vi "9149 FPGA VI.vi"() -> ()   [LabVIEW 2017]
uses:
  <vilib>/Platform/TimedLoop/XDataNode/timing_clust.ctl
  <vilib>/Platform/TimedLoop/XDataNode/nitl_modes.ctl
  <vilib>/Platform/TimedLoop/XDataNode/wakeup.ctl
  <vilib>/rvi/Emulation/niFpgaGetClockAttributes.vi
  <vilib>/rvi/Emulation/niFpgaSctlEmulationGetInTimedLoop.vi
  <vilib>/rvi/Emulation/niFpgaEmulationReportErrorSimple.vi
  <vilib>/rvi/eio/common/nirviEmuTemplateMethod_errors.vi
  <vilib>/rvi/Emulation/niFpgaEmulationIsFPGAContextNoSignature.vi
  <vilib>/rvi/errors/niFpgaSetErrorForExecOnDevCompSimple.vi
  <vilib>/rvi/eio/common/nirviEmuReportErrorAndStop.vi
  <vilib>/rvi/DataTransferAndStorage/Container/Common/niFpgaContainerGetUniqueNameForEmu.vi
  <vilib>/rvi/FIFO/Fifo_Resource/nirvififoEmulationSetSize.vi
  <vilib>/rvi/FIFO/Fifo_Resource/nirviFifoEmulationQueueMgr.vi
  <instcachedir>/0/nirviFifoEmulationQueueMgr_E5CAEC123FF24DC58D834DCA3CDAA9B5.lvgen/nirviFifoEmulationQueueMgr_E5CAEC123FF24DC58D834DCA3CDAA9B5_008.vi
  <vilib>/rvi/FIFO/Fifo_Resource/nirvififoEmulationDetermineInputValidOut.vi
  <vilib>/rvi/FIFO/Fifo_Resource/nirvififoEmulationCreateLock.vi
  <vilib>/rvi/Emulation/niFpgaProcessEmulError.vi
  <vilib>/rvi/FIFO/Fifo_Resource/nirvififoEmulationObtainLock.vi
  <vilib>/rvi/FIFO/Fifo_Resource/nirvififoEmulationReleaseLock.vi
  <vilib>/rvi/occurrence/nirviWaitOnOccurrenceBase.vi
  <vilib>/rvi/errors/nirviReportUnexpectedCaseInternalError.vi
  <vilib>/rvi/errors/nirviReportUnexpectedCaseInternalError (U32).vi
  <vilib>/rvi/Emulation/niFpgaCriticalErrorInLSC.vi
  <vilib>/Utility/error.llb/Clear Errors.vi
  <vilib>/rvi/interface/RandomDataEmulation/niFpgaRandomDataHandleErrors.vi
  <vilib>/eio/EIONode/EIONode.xnode
  <vilib>/rvi/DataTransferAndStorage/Container/XNode/niFpgaContainer.xnode
  <vilib>/rvi/FIFO/Fifo_Resource/nirvififoEmulationWrite.vi
  <vilib>/Platform/TimedLoop/XDataNode/XDataNode.xnode
  <vilib>/rvi/FIFO/Fifo_Resource/nirvififoEmulationRead.vi
  <vilib>/rvi/interface/RandomDataEmulation/nirviRandomDataFpgaReadWriteTemplate.vi
  <vilib>/Platform/TimedLoop/XDataNode/XDNodeRunTimeDep.lvlib
panel:
  out "Mod3_AI15_I32":i32
  out "Mod3_AI14_I32":i32
  out "Mod3_AI13_I32":i32
  out "Mod3_AI12_I32":i32
  out "Mod3_AI11_I32":i32
  out "Mod3_AI10_I32":i32
  out "Mod3_AI9_I32":i32
  out "Mod3_AI8_I32":i32
  out "Mod3_AI7_I32":i32
  out "Mod3_AI6_I32":i32
  out "Mod3_AI5_I32":i32
  out "Mod3_AI4_I32":i32
  out "TargetToHostLoopIterCount":i32
  out "TargetToHostLoopTimedOut":bool
  out "Mod6_U32":u32
  in  "Mod1_U32":u32
  in  "SlowDOLoop_Rate_us":u32=10000 caption="Count(uSec)"
  out "SlowDOLoop_Duration_ticks":u32
  in  "FastAILoop_Rate_us":u32=1000 caption="Count(uSec)"
  out "FastAILoop_Duration_ticks":u32
  out "Mod3_AI3_I32":i32
  out "Mod3_AI2_I32":i32
  out "Mod3_AI1_I32":i32
  out "Mod3_AI0_I32":i32
  out "SlowScanLoopTimedOut":bool
  out "SlowScanLoop_Duration_ticks":u32
  in  "SlowScanLoop_Rate_us":u32=10000 caption="Count(uSec)"
  in  "FastDO_Mod5_U8":u8
  out "FastDI_Mod8_U8":u8
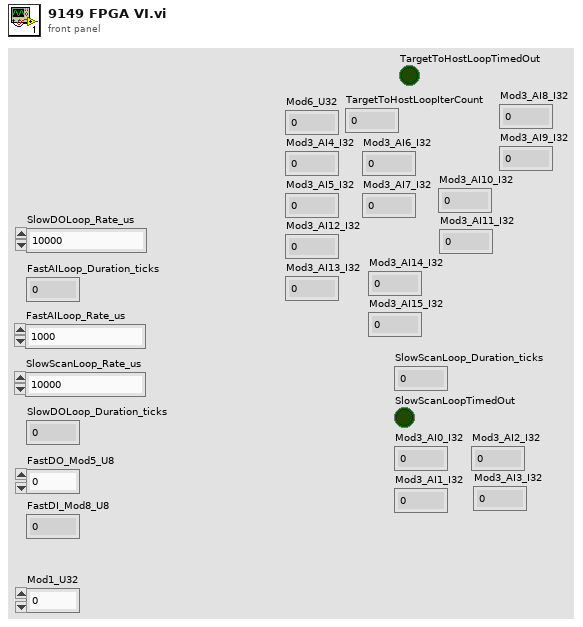
[diagram p1: front panel]
types:
  T1 = typedef "XDNodeRunTimeDep.lvlib/timing_clust.ctl" = cluster{"Expected End [f-1]":u64, "Actual End [f-1]":u64, "Finished Late? [f-1]":bool, "Expected End [i-1]":u64, "Actual End [i-1]":u64, "Finished Late? [i-1]":bool, "Expected Start [i]":u64, "Actual Start [i]":u64, "Expected Start [f]":u64, "Actual Start [f]":u64, "Source Name":string, "Structure Name":string, "Period":i64, "Deadline":i64, "Offset":i64, "Start":i64, "Priority":i32, "Timeout":i32, "Mode":T2, "Wakeup Reason":T3, "Error":errorcluster, "Source Type":string, "Secondary Source Type":string, "Global End Time":u64, "Global Start Time":u64, "Frame Duration":u64, "Iteration Duration":u64, "Assigned CPU":i32, "I/O Scan Engine Mode":u32}
  T2 = typedef "XDNodeRunTimeDep.lvlib/nitl_modes.ctl" = enum32{"No Change", "Process missed periods, maintain original phase", "Discard missed periods, maintain original phase", "Process missed periods, ignore original phase", "Discard missed periods, ignore original phase"}
  T3 = typedef "XDNodeRunTimeDep.lvlib/wakeup.ctl" = enum32{"Normal", "Aborted", "Asynchronous wakeup", "Timing source error", "Timed loop error", "Timeout"}
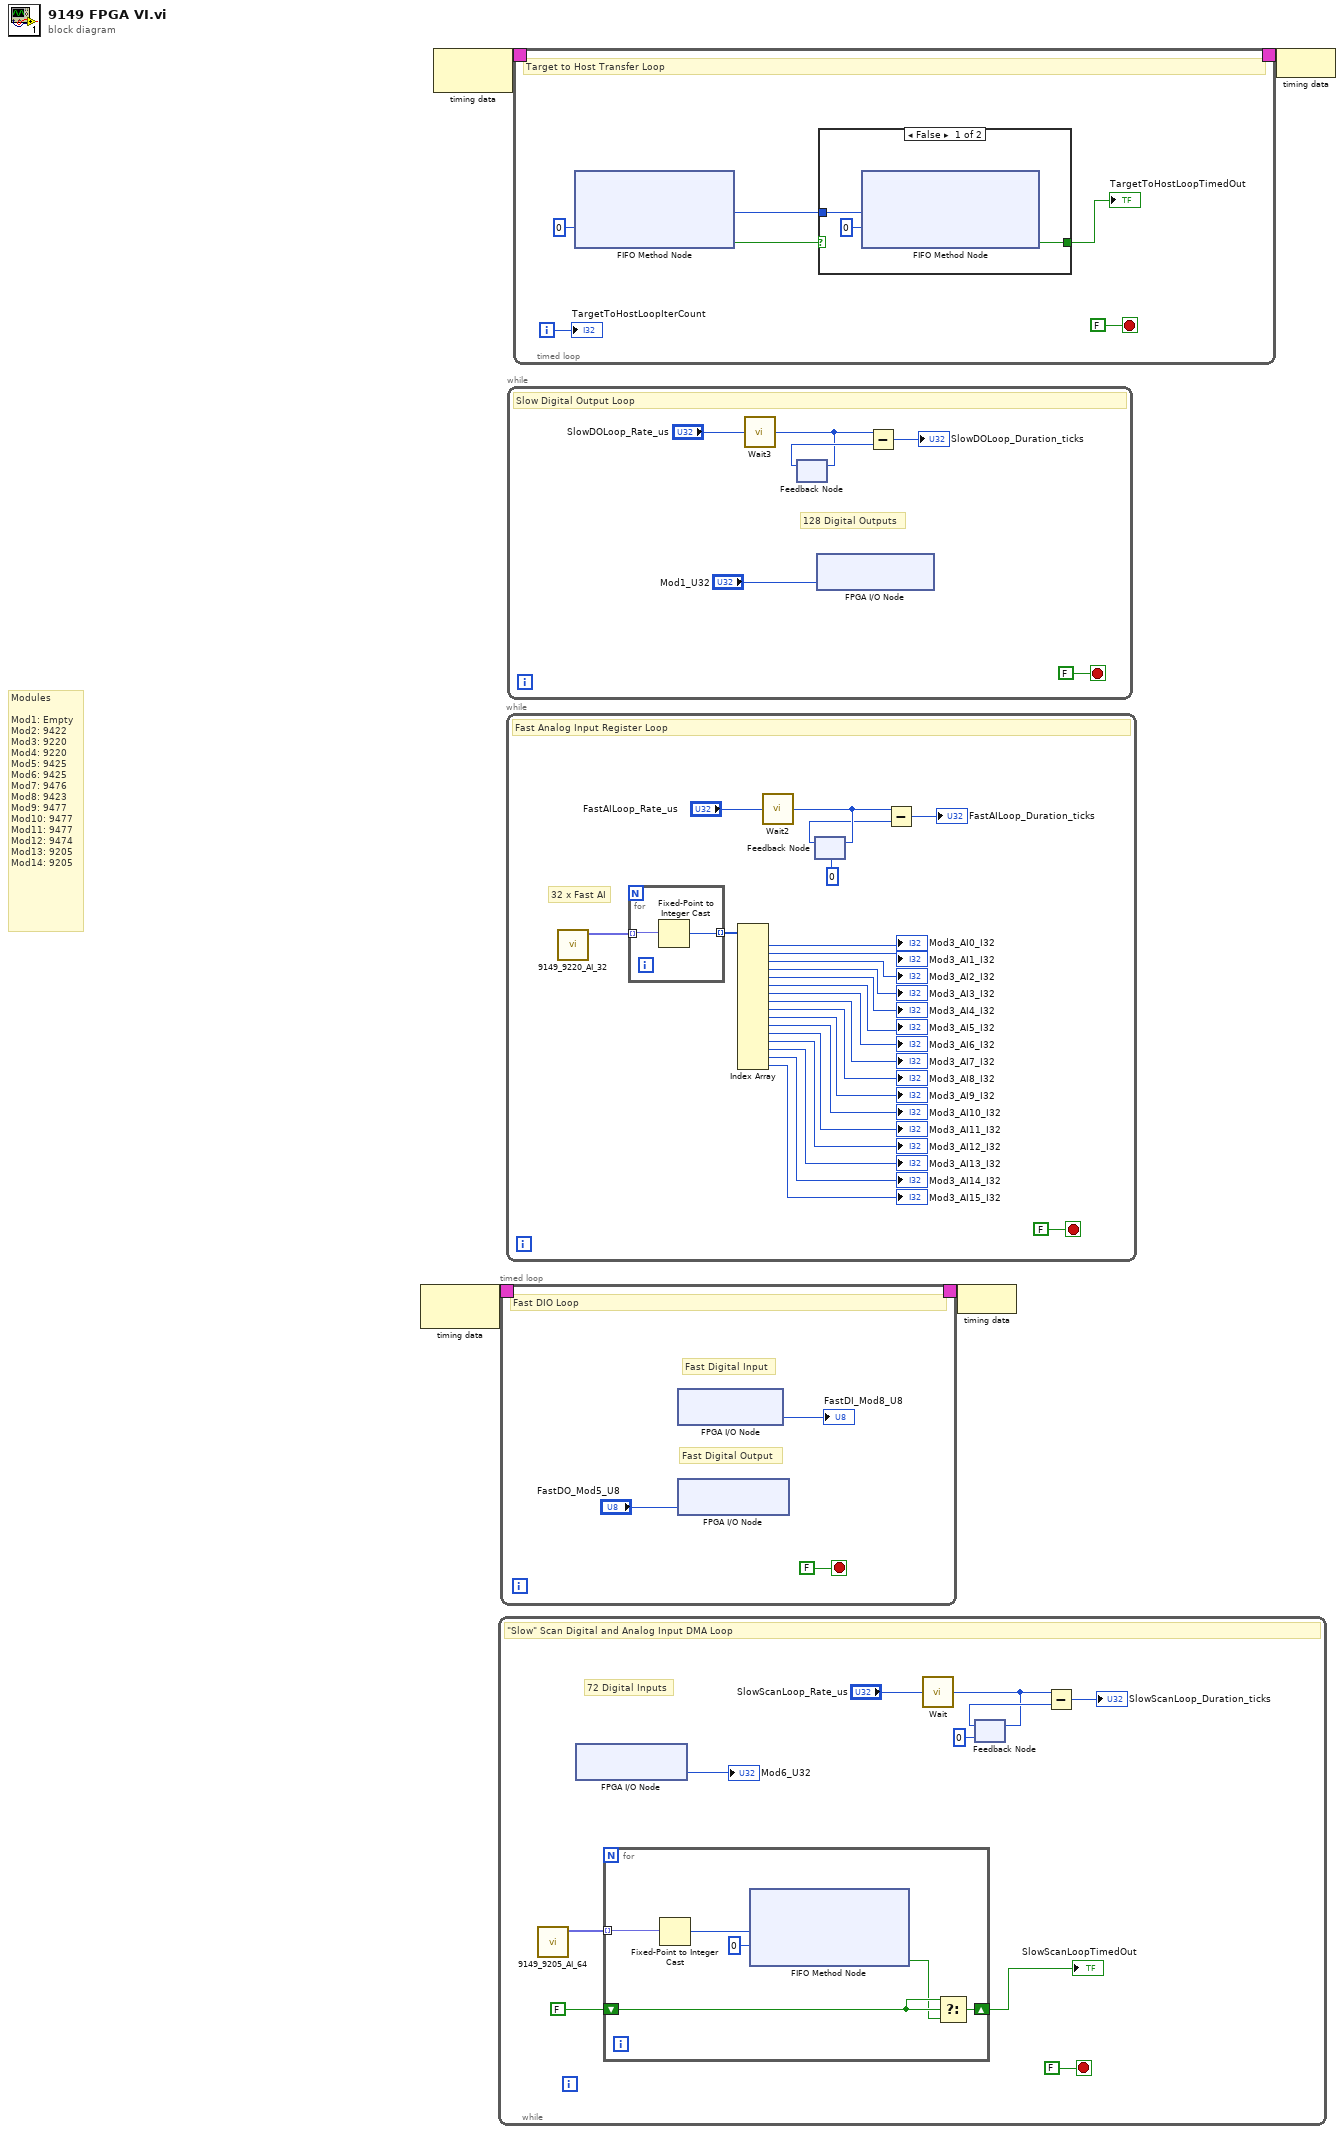
[diagram p0: block diagram]
diagram:
  # "Modules\n\nMod1: Empty\nMod2: 9422\nMod3: 9220\nMod4: 9220\nMod5: 9425\nMod6: 9425\nMod7: 9476\nMod8: 9423\nMod9: 9477\nMod10: 9477\nMod11: 9477\nMod12: 9474\nMod13: 9205\nMod14: 9205"
  n1 = node-c288() -> (w2:T1)  [unwired: 1 in]
  n2 = node-c288() -> (w4:T1)  [unwired: 1 in]
  n3 = while {
    stop <- FALSE stop-if-true
    # "72 Digital Inputs"
    # "\"Slow\" Scan Digital and Analog Input DMA Loop"
    n4 = call "9149_9205_AI_64.vi"() -> ("Array"=w7:fxp<+/-,26,5>[])  [unwired: 11 in]
    n5 = xnode "FPGA I/O Node"() -> ("Mod6/DI31:0"=→"Mod6_U32":u32)  [unwired: 1 in, 1 out]
    n6 = for {
      shift-right: [w18] -> w9
      shift-left: FALSE ("Timed Out?") -> [w20]
      tunnel: w7 -> [w17] mode=indexing
      n7 = Fixed-Point to Integer Cast(1:w17) -> (0:w16:i32)
      n8 = xnode ("FIFO Method Node")("Element"=w16, "Timeout"=0) -> ("Timed Out?"=w19:bool)  [unwired: 1 in, 1 out]
      n9 = Select(t=w20, s=w20, f=w19) -> (s? t:f=w18:bool)
    }
    "SlowScanLoopTimedOut" <- w9
    n10 = call "Wait"("Count(uSec)"="SlowScanLoop_Rate_us") -> ("Tick Count(uSec)"=w11:u32)
    n11 = feedback-in #1(w11) -> ()
    n12 = feedback #1(u32 0 ("Tick Count(uSec)")) -> (w12:u32)
    n13 = Subtract(x=w11, y=w12) -> (x-y=→"SlowScanLoop_Duration_ticks":u32)
  }
  n14 = timed-loop {
    timing: w2 -> [_]
    timing-out: [_] -> w1
    stop <- FALSE stop-if-true
    # "Fast Digital Output"
    # "Fast Digital Input"
    # "Fast DIO Loop"
    n15 = xnode "FPGA I/O Node"() -> ("Mod8/DI7:0"=→"FastDI_Mod8_U8":u8)  [unwired: 1 in, 1 out]
    n16 = xnode "FPGA I/O Node"("Mod5/DO7:0"="FastDO_Mod5_U8") -> ()  [unwired: 1 in, 1 out]
  }
  n17 = while {
    stop <- FALSE stop-if-true
    # "32 x Fast AI"
    # "Fast Analog Input Register Loop"
    n18 = call "9149_9220_AI_32.vi"() -> ("Array"=w48:fxp<+/-,24,5>[])  [unwired: 11 in]
    n19 = for {
      tunnel: w48 -> [w51] mode=indexing
      tunnel: [w50] -> w47 mode=indexing
      n20 = Fixed-Point to Integer Cast(1:w51) -> (0:w50:i32)
    }
    n21 = Index Array(array=w47) -> (element #1=→"Mod3_AI0_I32":i32, element #2=→"Mod3_AI1_I32":i32, element #3=→"Mod3_AI2_I32":i32, element #4=→"Mod3_AI3_I32":i32, element #5=→"Mod3_AI4_I32":i32, element #6=→"Mod3_AI5_I32":i32, element #7=→"Mod3_AI6_I32":i32, element #8=→"Mod3_AI7_I32":i32, element #9=→"Mod3_AI8_I32":i32, element #10=→"Mod3_AI9_I32":i32, element #11=→"Mod3_AI10_I32":i32, element #12=→"Mod3_AI11_I32":i32, element #13=→"Mod3_AI12_I32":i32, element #14=→"Mod3_AI13_I32":i32, element #15=→"Mod3_AI14_I32":i32, element #16=→"Mod3_AI15_I32":i32)  [unwired: 16 in]
    n22 = call "Wait2"("Count(uSec)"="FastAILoop_Rate_us") -> ("Tick Count(uSec)"=w41:u32)
    n23 = feedback #2(u32 0 ("Tick Count(uSec)")) -> (w40:u32)
    n24 = feedback-in #2(w41) -> ()
    n25 = Subtract(x=w41, y=w40) -> (x-y=→"FastAILoop_Duration_ticks":u32)
  }
  n26 = while {
    stop <- FALSE stop-if-true
    # "128 Digital Outputs"
    # "Slow Digital Output Loop"
    n27 = call "Wait3"("Count(uSec)"="SlowDOLoop_Rate_us") -> ("Tick Count(uSec)"=w55:u32)
    n28 = feedback #3() -> (w56:u32)  [unwired: 1 in]
    n29 = feedback-in #3(w55) -> ()
    n30 = xnode "FPGA I/O Node"("Mod1/DO31:0"="Mod1_U32") -> ()  [unwired: 1 in, 1 out]
    n31 = Subtract(x=w55, y=w56) -> (x-y=→"SlowDOLoop_Duration_ticks":u32)
  }
  n32 = timed-loop {
    timing: w4 -> [_]
    timing-out: [_] -> w3
    i -> [w59]
    stop <- FALSE stop-if-true
    # "Target to Host Transfer Loop"
    n33 = xnode ("FIFO Method Node")("Timeout"=0) -> ("Element"=w61:i32, "Timed Out?"=w63:bool)  [unwired: 1 in, 1 out]
    n34 = case shown="False" w63 {
      tunnel: w61 -> [w66 _]
      tunnel: [w64 _] -> w60
      frame False {
        n35 = xnode ("FIFO Method Node")("Element"=w66, "Timeout"=0) -> ("Timed Out?"=w64:bool)  [unwired: 1 in, 1 out]
      }
      frame True {
      }
    }
    "TargetToHostLoopTimedOut" <- w60
    "TargetToHostLoopIterCount" <- w59
  }
  n36 = node-c288(w1) -> ()
  n37 = node-c288(w3) -> ()
